vi "niHWS New Wfm Reference.vi"(7 "compression level (0:none)":i32 min=0 max=9 step=1, 8 "error in (no error)":errorcluster, 9 "waveform name (empty)":string, 10 "group name (empty)":string, 11 "file handle in":u32) -> (0 "error out":errorcluster, 2 "waveform reference":u32, 3 "file handle out":u32)   [LabVIEW 2011]
doc: "Creates a new waveform in the specified group and returns a reference to it.\n\nWaveforms are identified by reference for purposes of setting and getting waveform attributes and reading and writing data."
uses:
  nihwsu.dll
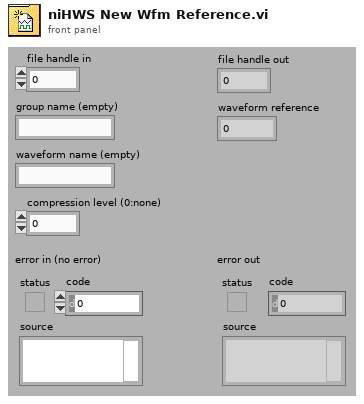
[diagram p1: front panel]
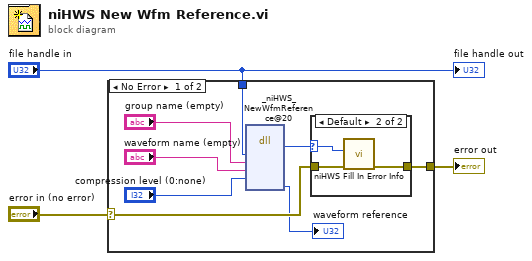
[diagram p0: block diagram]
diagram:
  n1 = case shown="No Error" "error in (no error)" {
    selector: "error in (no error)" -> [w6 w16]
    tunnel: [w8 w16] -> w2
    tunnel: "file handle in" -> [w5 _]
    frame No Error {
      n2 = dll-call lib="nihwsu.dll" fn="_niHWS_NewWfmReference@20"("fileHandle"=w5, "groupName"="group name (empty)", "wfmName"="waveform name (empty)", "compressionLevel"="compression level (0:none)") -> (w7:i32, "wfmRef"=→"waveform reference":u32)  [unwired: 8 in, 2 out]
      n3 = case shown="Default" w7 {
        selector: w7 -> [_ w13]
        tunnel: [w12 w14] -> w8
        tunnel: w6 -> [w12 w15]
        frame 0 {
        }
        frame Default {
          n4 = call "niHWS Fill In Error Info.vi"("error in (no error)"=w15, "status code"=w13) -> ("error out"=w14:errorcluster)  [unwired: 9 in]
        }
      }
    }
    frame Error {
    }
  }
  "error out" <- w2
  "file handle out" <- "file handle in"
